vi "Count Lines.vi"(10 "String Input":string) -> (2 "Number of Lines":i32)   [LabVIEW 2017]
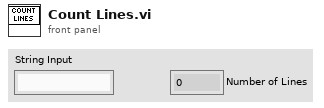
[diagram p1: front panel]
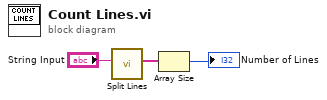
[diagram p0: block diagram]
diagram:
  n1 = call "Split Lines.vi"("String In"="String Input") -> ("Lines Out"=w1:string[])  [unwired: 10 in]
  n2 = Array Size(array=w1) -> (size(s)=→"Number of Lines":i32)
